vi "AI Base Globals.vi"() -> ()   [LabVIEW 2023, in "LabVIEW AI Base.lvlib"]
uses:
  LabVIEW AI Base.lvlib
  <vilib>/httpClient/ClientHandle.ctl
  <vilib>/httpClient/LabVIEWHTTPClient.lvlib
panel:
  in  "Tab Control":enum32{"Python Settings", "LLM Settings"}(tab)
  out "Python Session":refnum<k35>
  in  "venv path":path=path "C:/dev/gaoruhao/labview-ai"
  in  "Anaconda path":path=path "C:/ProgramData/miniforge3"
  in  "Python version":string="3.10"
  in  "conda env name":string="ai"
  out "Http Client Handle":T1
  in  "OpenAI API URL":string="https://openrouter.ai/api/v1" caption="OpenAI API URL (e.g. OpenRouter, LM Studio)"
  in  "API Key":string="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"
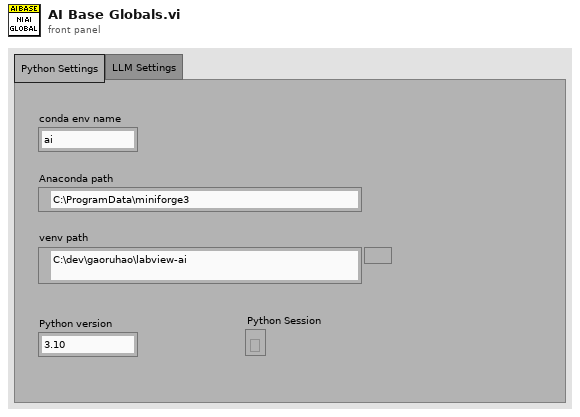
[diagram p1: front panel]
types:
  T1 = typedef "LabVIEWHTTPClient.lvlib/ClientHandle.ctl" = refnum<k1>
diagram:
